vi "Display_message.vi"(2 "Time to display message":u32, 3 "Message":string) -> (0 "VI name":string)   [LabVIEW 2017]
panel:
  out "Message Display":string
  out "Last Written to:":string
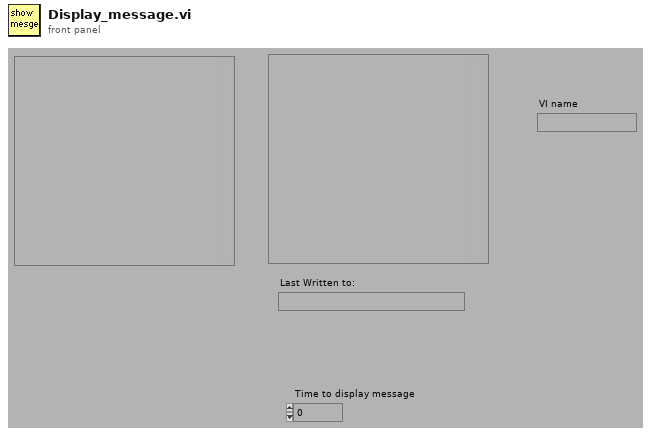
[diagram p1: front panel]
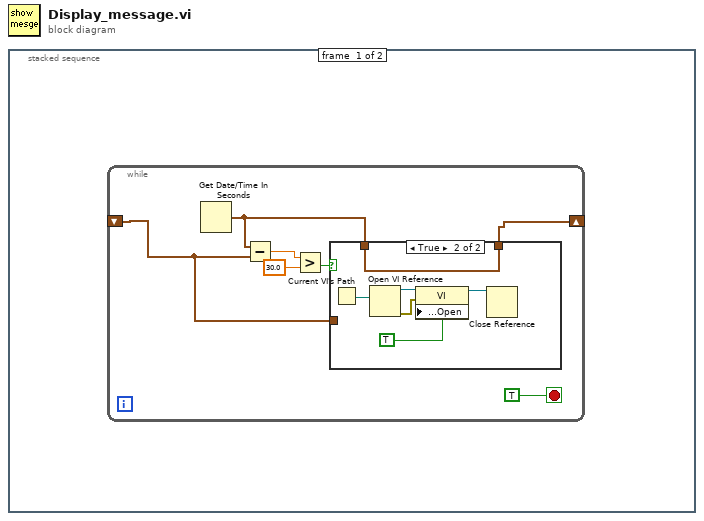
[diagram p0: block diagram]
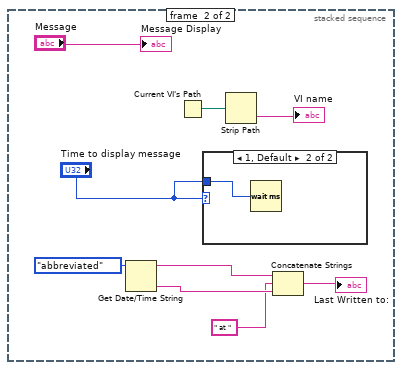
[diagram p3: hidden frame]
diagram:
  n1 = stacked-sequence {
    frame #0 {
      n2 = while {
        shift-right: [w3] -> _
        shift-left: _ -> [w1]
        stop <- TRUE stop-if-true
        n3 = Get Date/Time In Seconds() -> (seconds since 1Jan1904=w2:timestamp)
        n4 = Subtract(x=w2, y=w1) -> (x-y=w7:dbl)
        n5 = Greater?(x=w7, y=30.0) -> (0:w4:bool)
        n6 = case shown="True" w4 {
          tunnel: [w8 w9] -> w3
          tunnel: w2 -> [_ w9]
          tunnel: w1 -> [w8 _]
          frame False {
          }
          frame True {
            n7 = Current VI's Path() -> (path=w14:path)
            n8 = Open VI Reference(vi path=w14) -> (vi reference=w13:refnum<vi>, error out=w12:errorcluster)  [unwired: 1 in, 4 out]
            n9 = property class="VI"(reference=w13, error in=w12, "Front Panel Window:Open"=TRUE) -> (reference out=w11:refnum<vi>)  [unwired: 1 out]
            n10 = Close Reference(reference=w11) -> ()  [unwired: 1 in, 1 out]
          }
        }
      }
    }
    frame #1 {
      n11 = Get Date/Time String(date format (0)=enum16{"short", "long", "abbreviated"}."abbreviated") -> (date string=w21:string, time string=w20:string)  [unwired: 2 out]
      n12 = Current VI's Path() -> (path=w23:path)
      n13 = case shown="1, Default" "Time to display message" {
        tunnel: "Time to display message" -> [_ w24]
        frame 0 {
        }
        frame 1, Default {
          n14 = Wait (ms)(milliseconds to wait=w24) -> ()  [unwired: 1 out]
        }
      }
      n15 = Strip Path(path=w23) -> (name=→"VI name":string)  [unwired: 1 out]
      n16 = Concatenate Strings(w21, " at ", w20) -> (→"Last Written to:":string)
      "Message Display" <- "Message"
    }
  }
